vi "ARC_Comm Application Exit.vi"(8 "error in (no error)":errorcluster, 10 "exit at development? (F)":bool, 11 "This VI":refnum<vi>) -> (0 "error out":errorcluster)   [LabVIEW 2016]
doc: "在编译环境下，此VI将应用程序退出，在编辑环境下，如果exit at development?为True，退出LabVIEW，否则不操作"
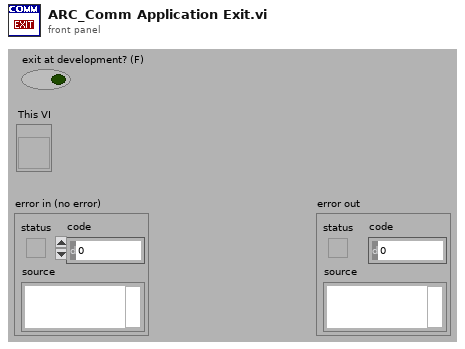
[diagram p1: front panel]
types:
  T1 = enum32{"invalid app kind", "Development System", "Run Time System", "Student Edition", "Embedded LabVIEW", "Evaluation", "Custom"}
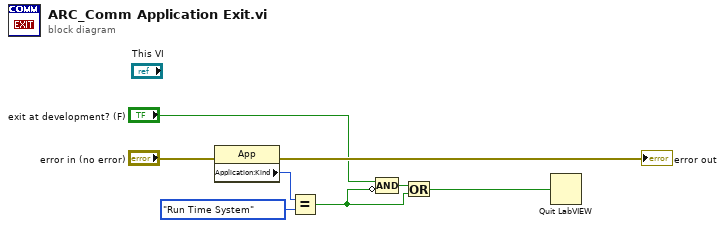
[diagram p0: block diagram]
diagram:
  n1 = property class="App"(error in="error in (no error)") -> (error out=→"error out":errorcluster, "Application:Kind"=w8:T1)  [unwired: 1 in, 1 out]
  n2 = Equal?(x=w8, y=T1."Run Time System") -> (x = y?=w5:bool)
  n3 = Compound Arithmetic op=AND("exit at development? (F)", invert w5) -> (w6:bool)
  n4 = Or(x=w6, y=w5) -> (x .or. y?=w4:bool)
  n5 = Quit LabVIEW(quit? (T)=w4) -> ()
